vi "Do.vi"(8 "error in (no error)":errorcluster, 10 "Actor in":refnum<class "Actor.lvclass">, 11 "Wait on Message Msg":refnum<class "Wait on Message Msg.lvclass">) -> (0 "error out":errorcluster, 2 "Actor out":refnum<class "Actor.lvclass">)   [LabVIEW 2019, in "ConnectionReader.lvlib" / "Wait on Message Msg.lvclass"]
doc: "This VI delivers the message to the actor by calling the appropriate method(s) on the actor."
uses:
  <vilib>/gpm_packages/@cs/Network-interface/Source/ConnectionReader/ConnectionReader Messages/Wait on Message Msg/Wait on Message Msg.lvclass
  C:/Program Files/National Instruments/LabVIEW 2019/vi.lib/ActorFramework/Message/Message.lvclass
  <vilib>/ActorFramework/Actor/Actor.lvclass
  <vilib>/gpm_packages/@cs/Network-interface/Source/ConnectionReader/ConnectionReader/ConnectionReader.lvclass
  C:/Program Files/National Instruments/LabVIEW 2019/vi.lib/gpm_packages/@cs/Network-interface/Source/Logged Actor/LoggedActor.lvclass
  C:/Program Files/National Instruments/LabVIEW 2019/vi.lib/ActorFramework/Actor/Actor.lvclass
  <vilib>/gpm_packages/@cs/Network-interface/Source/ConnectionReader/ConnectionReader/ConnectionReader.lvclass/ConnectionReader.ctl
  <vilib>/gpm_packages/@cs/Network-interface/Source/Logged Actor/LoggedActor.lvclass/LoggedActor.ctl
  <vilib>/gpm_packages/@cs/event-logger/Source/Composed Log/LoggerReference/LoggerReference.lvclass/LoggerReference.ctl
  <vilib>/ActorFramework/Actor/Actor.lvclass/Actor.ctl
  <vilib>/ActorFramework/Message Enqueuer/Message Enqueuer.lvclass/Message Enqueuer.ctl
  <vilib>/gpm_packages/@cs/Network-interface/Source/Logged Actor/Log Session Event.vi
  <vilib>/ActorFramework/Actor/Read Self Enqueuer.vi
  <vilib>/gpm_packages/@cs/event-logger/Source/Composed Log/LoggerReference/Log Event.vi
  <vilib>/ActorFramework/Message Enqueuer/Init from Existing Queue.vi
  <vilib>/gpm_packages/@cs/event-logger/Source/Composed Log/LoggerReference/Log.vi
  <vilib>/gpm_packages/@cs/event-logger/Source/Composed Log/LoggerReference/Get Valid Event Time.vi
  <vilib>/gpm_packages/@cs/event-logger/Source/Composed Log/LoggerReference/Remove Stale Logs.vi
  <vilib>/ActorFramework/Message Priority Queue/Priority Enqueue.vi
  <vilib>/gpm_packages/@cs/Network-interface/Source/MessagingInterfaces/IPacket/IPacket.lvclass
  <vilib>/ActorFramework/Message Enqueuer/Message Enqueuer.lvclass
  <vilib>/gpm_packages/@cs/Network-interface/Source/MessagingInterfaces/IReadStrategy/IReadStrategy.lvclass
  <vilib>/gpm_packages/@cs/Network-interface/Source/MessagingInterfaces/IMessageReturnPolicy/IMessageReturnPolicy.lvclass
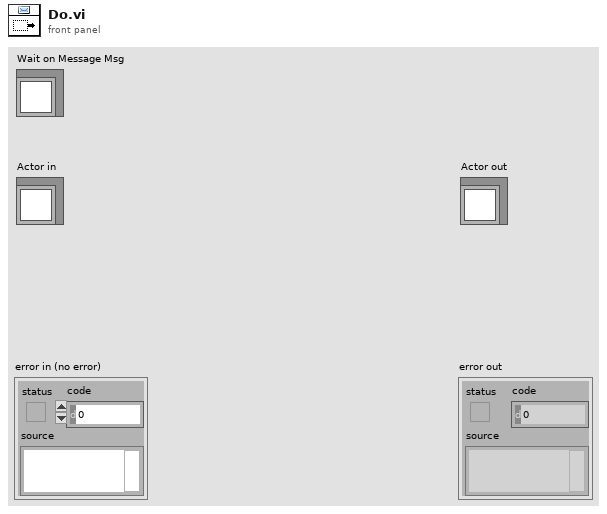
[diagram p1: front panel]
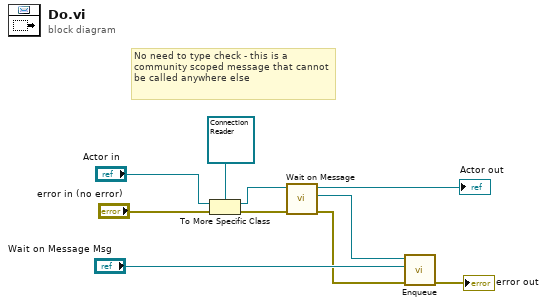
[diagram p0: block diagram]
diagram:
  # "No need to type check - this is a community scoped message that cannot be called anywhere else"
  n1 = To More Specific Class(target class=refnum<class "ConnectionReader.lvclass"> refnum ("Actor in"), reference="Actor in", error in="error in (no error)") -> (specific class reference=w6:refnum<class "ConnectionReader.lvclass">, error out=w9:errorcluster)
  n2 = call <vilib>:"Wait on Message.vi"("error in (no error)"=w9, "ConnectionReader in"=w6) -> ("error out"=w4:errorcluster, "Self Enqueuer"=w2:refnum<class "Message Enqueuer.lvclass">, "ConnectionReader out"=→"Actor out":refnum<class "ConnectionReader.lvclass">)  [unwired: 7 in]
  n3 = call <vilib>:"Enqueue.vi"("error in (no error)"=w4, "Message"="Wait on Message Msg", "Message Enqueuer in"=w2) -> ("error out"=→"error out":errorcluster)  [unwired: 7 in, 1 out]
